vi "Edge Detector.vi"(10 "Mode":enum16{"Rising", "Falling", "Any"}(ring), 11 "Input":bool) -> (3 "Output":bool)   [LabVIEW 2016, in "memLib.lvlib"]
uses:
  <vilib>/FRCT Team# 3937  Breakaway/Memory Library/memLib.lvlib
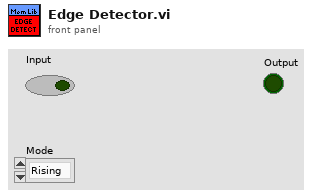
[diagram p1: front panel]
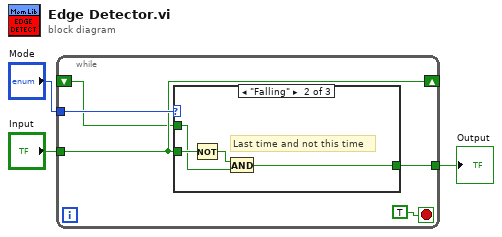
[diagram p0: block diagram]
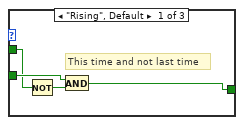
[diagram p2: hidden frame]
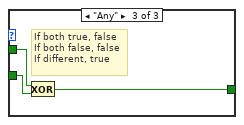
[diagram p3: hidden frame]
diagram:
  n1 = while {
    tunnel: "Mode" -> [w8]
    tunnel: "Input" -> [w6]
    shift-right: [w6] -> _
    shift-left: _ -> [w5]
    tunnel: [w4] -> w1
    stop <- TRUE stop-if-true
    n2 = case shown="\"Falling\"" w8 {
      tunnel: w6 -> [w12 w16 w18]
      tunnel: w5 -> [w11 w13 w19]
      tunnel: [w9 w15 w17] -> w4
      frame "Rising", Default {
        # "This time and not last time"
        n3 = Not(x=w11) -> (.not. x?=w10:bool)
        n4 = And(x=w12, y=w10) -> (x .and. y?=w9:bool)
      }
      frame "Falling" {
        # "Last time and not this time"
        n5 = Not(x=w16) -> (.not. x?=w14:bool)
        n6 = And(x=w14, y=w13) -> (x .and. y?=w15:bool)
      }
      frame "Any" {
        # "If both true, false\nIf both false, false\nIf different, true"
        n7 = Exclusive Or(1:w18, 2:w19) -> (0:w17:bool)
      }
    }
  }
  "Output" <- w1
